vi "ManageSaving.vi"(8 "error in (no error)":errorcluster, 10 "Save Data":T2, 11 "Saving Thread Data in":T1) -> (0 "error out":errorcluster, 3 "Saving Thread Data out":T1)   [LabVIEW 2019]
uses:
  Typedefs/Saving Thread/#cluster_SavingThreadData.ctl
  Typedefs/Saving Thread/#cluster_SaveData.ctl
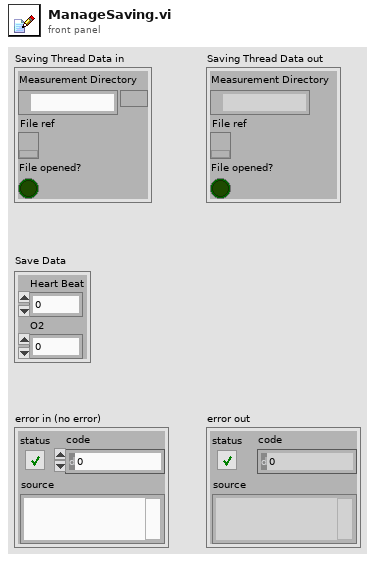
[diagram p1: front panel]
types:
  T1 = typedef "#cluster_SavingThreadData.ctl" = cluster{"Measurement Directory":path, "File ref":refnum<k34>, "File opened?":bool}
  T2 = typedef "#cluster_SaveData.ctl" = cluster{"Heart Beat":dbl, "O2":dbl}
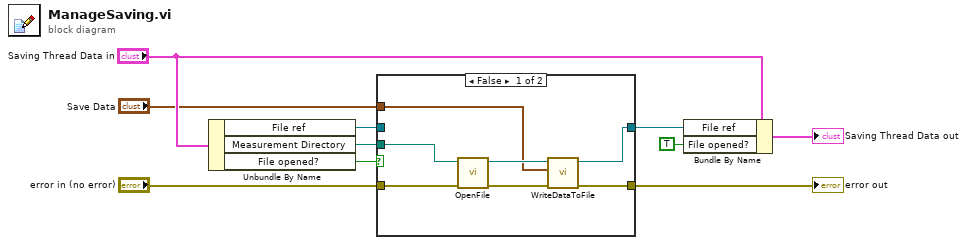
[diagram p0: block diagram]
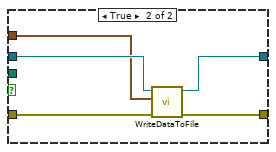
[diagram p2: hidden frame]
diagram:
  n1 = Unbundle By Name("Saving Thread Data in") -> ("File ref"=w7:refnum<k34>, "Measurement Directory"=w8:path, "File opened?"=w9:bool)
  n2 = case shown="False" w9 {
    tunnel: w8 -> [w15 _]
    tunnel: w7 -> [_ w22]
    tunnel: "error in (no error)" -> [w14 w21]
    tunnel: [w17 w20] -> w5
    tunnel: [w16 w19] -> w4
    tunnel: "Save Data" -> [w11 w18]
    frame False {
      n3 = call "OpenFile.vi"("error in (no error)"=w14, "Measurement Directory"=w15) -> ("error out"=w13:errorcluster, "File ref out"=w12:refnum<k34>)  [unwired: 8 in]
      n4 = call "WriteDataToFile.vi"("error in (no error)"=w13, "Save Data"=w11, "File ref in"=w12) -> ("error out"=w17:errorcluster, "File ref out"=w16:refnum<k34>)  [unwired: 7 in]
    }
    frame True {
      n5 = call "WriteDataToFile.vi"("error in (no error)"=w21, "Save Data"=w18, "File ref in"=w22) -> ("error out"=w20:errorcluster, "File ref out"=w19:refnum<k34>)  [unwired: 7 in]
    }
  }
  "error out" <- w5
  n6 = Bundle By Name(cluster="Saving Thread Data in", "File ref"=w4, "File opened?"=TRUE) -> (→"Saving Thread Data out":T1)
